vi "ROS_Topic_Close.vi"(0 "error in":errorcluster, 2 "ROS in":T1={"topic port"=0, "Node"="", "topic"="", "type"="", "node port"=0, "error "={"status"=FALSE, "code"=0, "source"=""}, "Direction"=enum."Node", "Update (ms)"=1, "FIFO size"=1}, 3 "node":string) -> (1 "error out":errorcluster)   [LabVIEW 2016]
doc: "Closes a topic. If no topic is defined, it will close all topics and all nodes."
uses:
  SubVIs/_ROSControl.ctl
  SubVIs/_ROSDirection.ctl
  ROS_Test1/UnicornRIO1/ROS for LabVIEW/home/lvuser/natinst/bin/user.lib/ROS for LabVIEW Software/ROS/Code/_ROSDefinition.vi
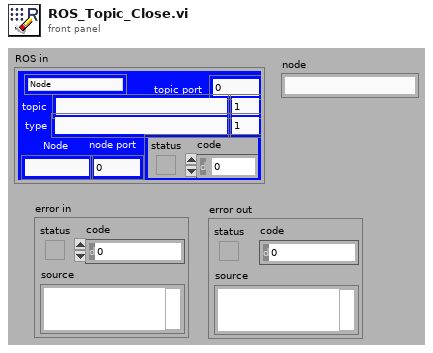
[diagram p1: front panel]
types:
  T1 = typedef "_ROSControl.ctl" = cluster{"topic port":u16, "Node":string, "topic":string, "type":string, "node port":u16, "error ":errorcluster, "Direction":T2, "Update (ms)":u16, "FIFO size":u16}
  T2 = typedef "_ROSDirection.ctl" = enum16{"Node", "Publisher", "Subscriber", "ServiceClient", "ServiceProvider"}
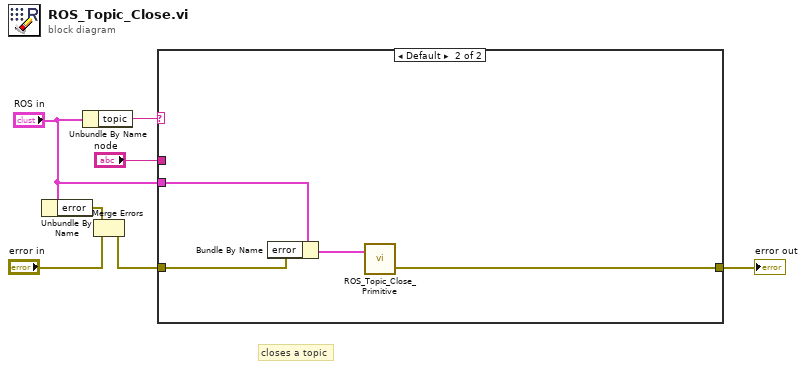
[diagram p0: block diagram]
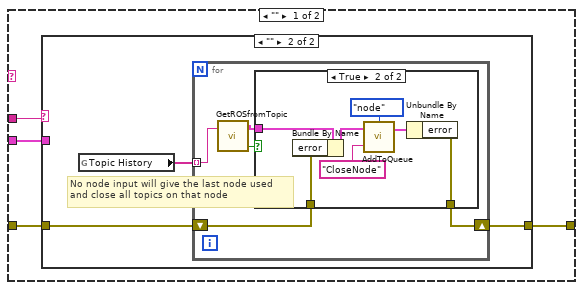
[diagram p2: hidden frame]
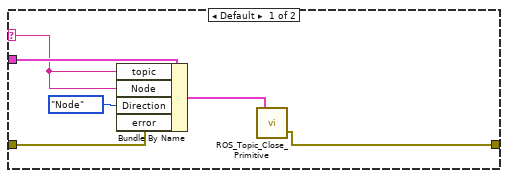
[diagram p3: hidden frame]
diagram:
  # "closes a topic"
  n1 = Unbundle By Name("ROS in") -> ("error"=w3:errorcluster)
  n2 = Unbundle By Name("ROS in") -> ("topic"=w6:string)
  n3 = Merge Errors(w3, "error in") -> (w1:errorcluster)
  n4 = case shown="Default" w6 {
    tunnel: w1 -> [w11 w36]
    tunnel: "ROS in" -> [w8 w35]
    tunnel: [w10 w37] -> w7
    tunnel: "node" -> [w9 _]
    frame "" {
      n5 = case shown="\"\"" w9 {
        selector: w9 -> [w13 _]
        tunnel: w11 -> [w12 w19]
        tunnel: [w14 w18] -> w10
        tunnel: w8 -> [w17 _]
        frame Default {
          n6 = Bundle By Name(cluster=w17, "topic"=w13, "Node"=w13, "Direction"=_ROSDirection."Node", "error"=w12) -> (w15:T1)
          n7 = call "ROS_Topic_Close_Primitive.vi"("ROS in"=w15) -> ("error out"=w14:errorcluster)  [unwired: 2 in]
        }
        frame "" {
          # "No node input will give the last node used\nand close all topics on that node"
          n8 = global read "_ROSDefinition.vi" "Topic History"() -> (w20:string[])
          n9 = for {
            tunnel: w20 -> [w23] mode=indexing
            shift-right: [w24] -> w18
            shift-left: w19 -> [w25]
            n10 = call "GetROSfromTopic.vi"("Topic"=w23) -> ("ROS"=w21:T1, "Node?"=w22:bool)  [unwired: 1 in, 1 out]
            n11 = case shown="True" w22 {
              tunnel: w25 -> [w26 w32]
              tunnel: [w26 w28] -> w24
              tunnel: w21 -> [_ w31]
              frame False {
              }
              frame True {
                n12 = Bundle By Name(cluster=w31, "error"=w32) -> (w30:T1)
                n13 = call "AddToQueue.vi"("Cmd"="CloseNode" ("format string"), "ROS"=w30, "Type"=enum16{"topic", "node", "ToFIFO", "ToWrite"}."node") -> ("ROS out"=w29:T1)  [unwired: 2 in]
                n14 = Unbundle By Name(w29) -> ("error"=w28:errorcluster)
              }
            }
          }
        }
      }
    }
    frame Default {
      n15 = Bundle By Name(cluster=w35, "error"=w36) -> (w34:T1)
      n16 = call "ROS_Topic_Close_Primitive.vi"("ROS in"=w34) -> ("error out"=w37:errorcluster)  [unwired: 2 in]
    }
  }
  "error out" <- w7
